vi "ChooseEstimation.vi"(6 "Time":enum16{"Azul", "Amarelo"}(ring) caption="Enum", 10 "Detection Frame Kalman":T1 {"robots_blue"."height" format="%+4.3f"; "robots_blue"."pixel_y" format="%+4.3f"; "robots_blue"."pixel_x" format="%+4.3f"; "robots_blue"."orientation" format="%+4.3f"; "robots_blue"."y" format="%+4.3f"; "robots_blue"."confidence" format="%4.3f"; "robots_blue"."x" format="%+4.3f"; "robots_yellow"."height" format="%+4.3f"; "robots_yellow"."pixel_y" format="%+4.3f"; "robots_yellow"."pixel_x" format="%+4.3f"; "robots_yellow"."orientation" format="%+4.3f"; "robots_yellow"."y" format="%+4.3f"; "robots_yellow"."confidence" format="%4.3f"; "robots_yellow"."x" format="%+4.3f"}, 11 "Detection Frame Kalman Vel Cmd":T1 {"robots_blue"."height" format="%+4.3f"; "robots_blue"."pixel_y" format="%+4.3f"; "robots_blue"."pixel_x" format="%+4.3f"; "robots_blue"."orientation" format="%+4.3f"; "robots_blue"."y" format="%+4.3f"; "robots_blue"."confidence" format="%4.3f"; "robots_blue"."x" format="%+4.3f"; "robots_yellow"."height" format="%+4.3f"; "robots_yellow"."pixel_y" format="%+4.3f"; "robots_yellow"."pixel_x" format="%+4.3f"; "robots_yellow"."orientation" format="%+4.3f"; "robots_yellow"."y" format="%+4.3f"; "robots_yellow"."confidence" format="%4.3f"; "robots_yellow"."x" format="%+4.3f"}) -> (2 "Detection Frame Out":T1 {"robots_blue"."height" format="%+4.3f"; "robots_blue"."pixel_y" format="%+4.3f"; "robots_blue"."pixel_x" format="%+4.3f"; "robots_blue"."orientation" format="%+4.3f"; "robots_blue"."y" format="%+4.3f"; "robots_blue"."confidence" format="%4.3f"; "robots_blue"."x" format="%+4.3f"; "robots_yellow"."height" format="%+4.3f"; "robots_yellow"."pixel_y" format="%+4.3f"; "robots_yellow"."pixel_x" format="%+4.3f"; "robots_yellow"."orientation" format="%+4.3f"; "robots_yellow"."y" format="%+4.3f"; "robots_yellow"."confidence" format="%4.3f"; "robots_yellow"."x" format="%+4.3f"})   [LabVIEW 2017]
uses:
  SSL Detection Frame.ctl
  SSL Detection Robot.ctl
  <vilib>/Analysis/Matrix/Datatypes/RealMatrix.ctl
  SSL Detection Ball.ctl
  <vilib>/Analysis/_algsub.llb/Real Vector Norm.vi
  <vilib>/ptbypt/NI_PtbyPt.lvlib
  <vilib>/Analysis/NI_AALPro.lvlib
  <vilib>/Analysis/Matrix/NI_Matrix.lvlib
panel:
  out "Enum":enum16{"Kalman Pure", "Kalman Vel Cmd"}(ring)
  out "norm 8":dbl
  out "norm 7":dbl
  out "norm 6":dbl
  out "norm 5":dbl
  out "Waveform Chart":cluster{"norm":dbl}(graph)
  out "norm 4":dbl
  out "norm 3":dbl
  out "norm 2":dbl
  out "norm":dbl
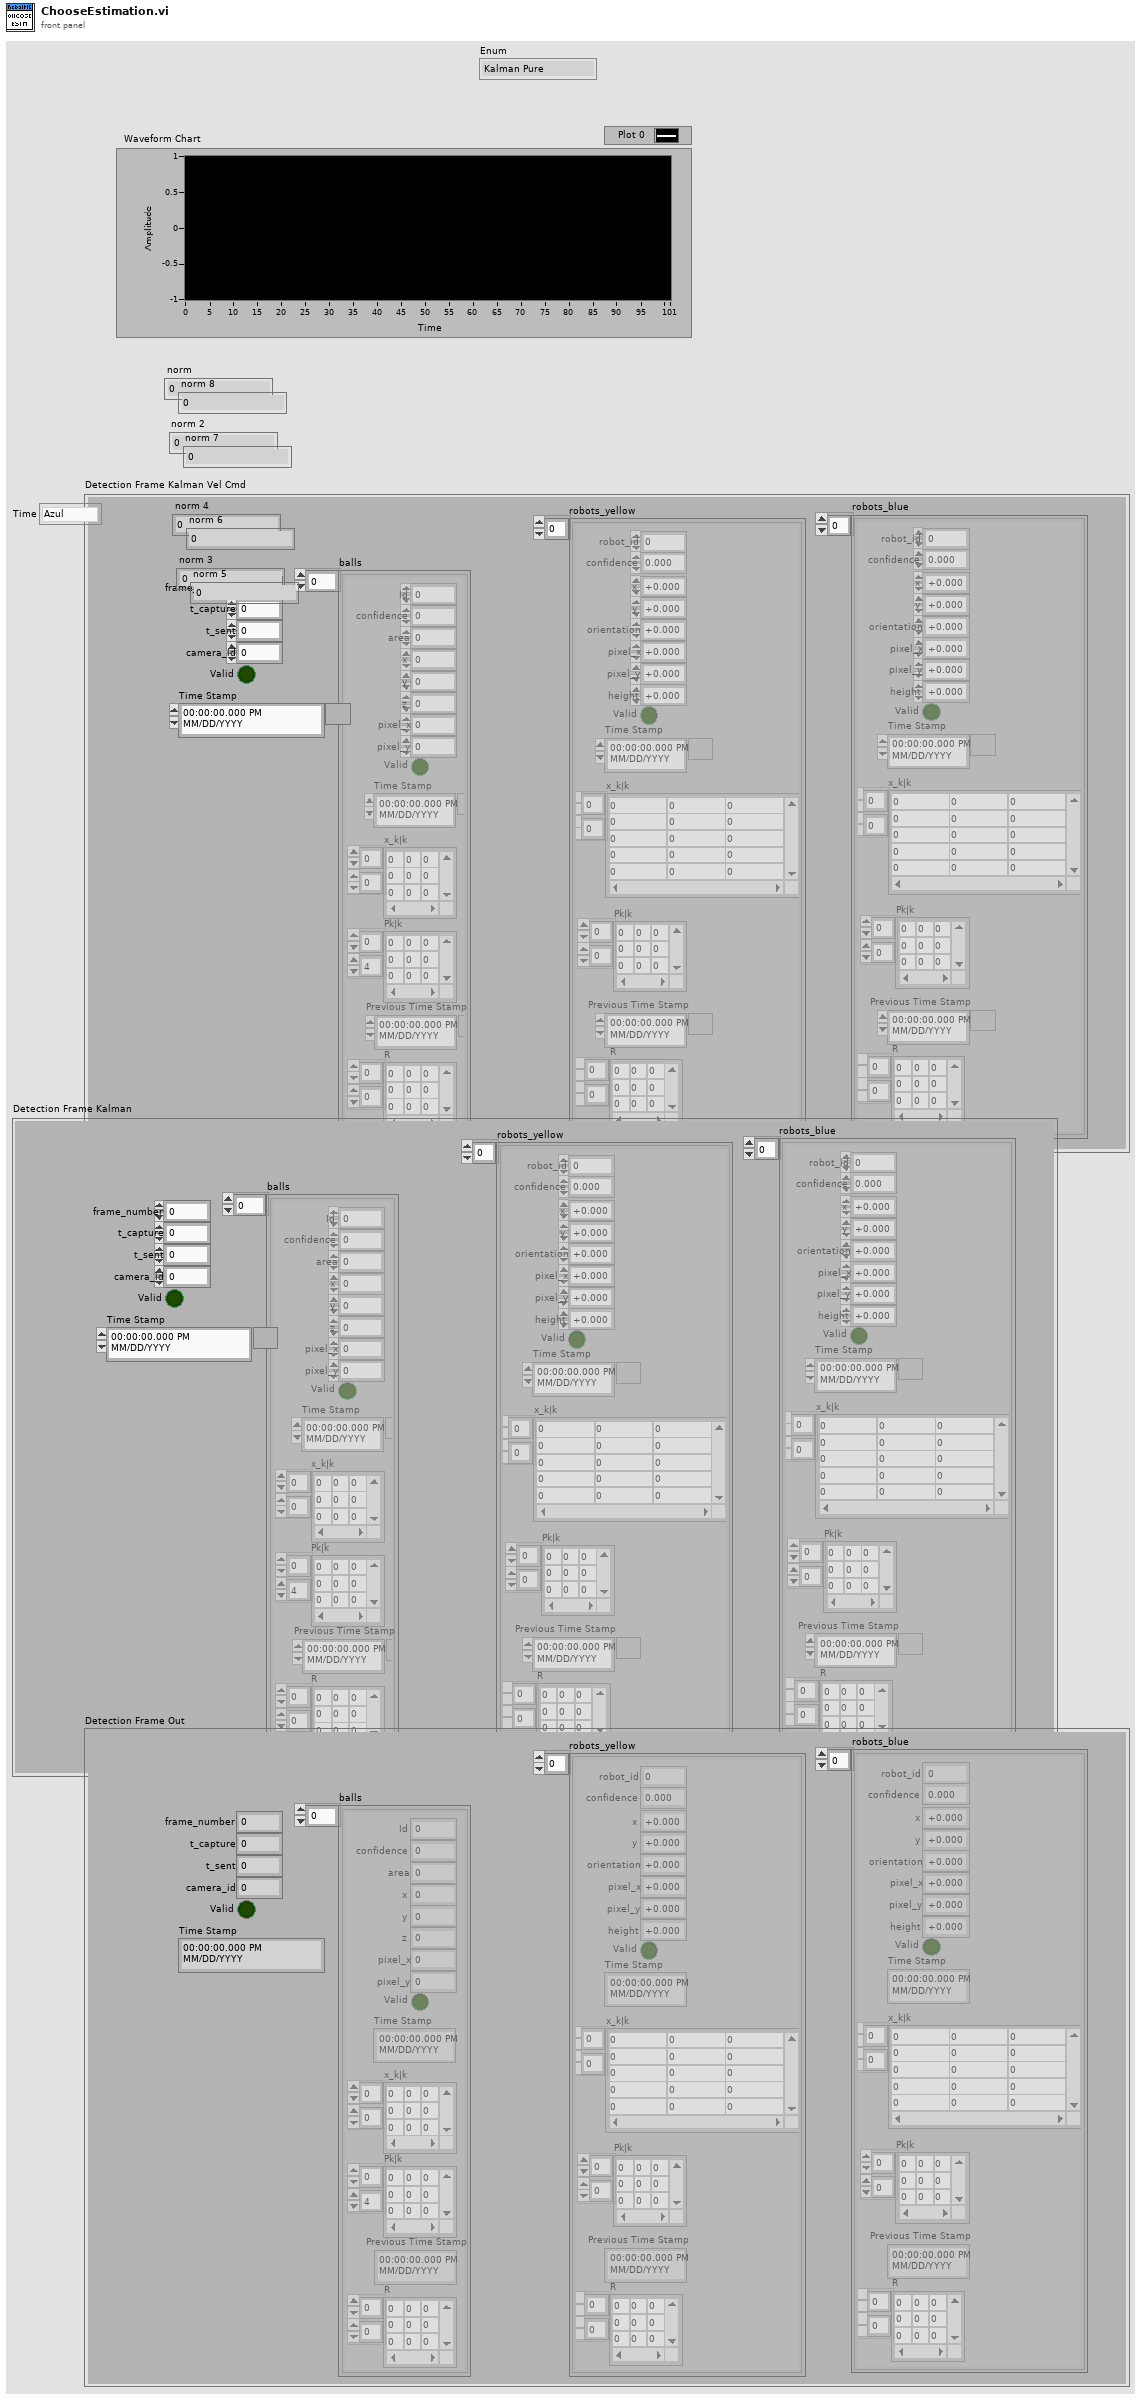
[diagram p1: front panel]
types:
  T1 = typedef "SSL Detection Frame.ctl" = cluster{"frame_number":u32, "t_capture":dbl, "t_sent":dbl, "camera_id":u32, "robots_yellow":T2[], "robots_blue":T2[], "balls":T4[], "Valid":bool, "Time Stamp":timestamp}
  T2 = typedef "SSL Detection Robot.ctl" = cluster{"x":sgl, "robot_id":u32, "confidence":sgl, "y":sgl, "orientation":sgl, "pixel_x":sgl, "pixel_y":sgl, "height":sgl, "Valid":bool, "Time Stamp":timestamp, "x_k|k":T3, "Pk|k":T3, "Previous Time Stamp":timestamp, "R":T3}
  T3 = typedef "NI_Matrix.lvlib/RealMatrix.ctl" = dbl[][]
  T4 = typedef "SSL Detection Ball.ctl" = cluster{"x":sgl, "area":u32, "confidence":sgl, "y":sgl, "z":sgl, "pixel_x":sgl, "pixel_y":sgl, "Valid":bool, "Time Stamp":timestamp, "x_k|k":T3, "Pk|k":T3, "Id":u32, "Previous Time Stamp":timestamp, "R":T3}
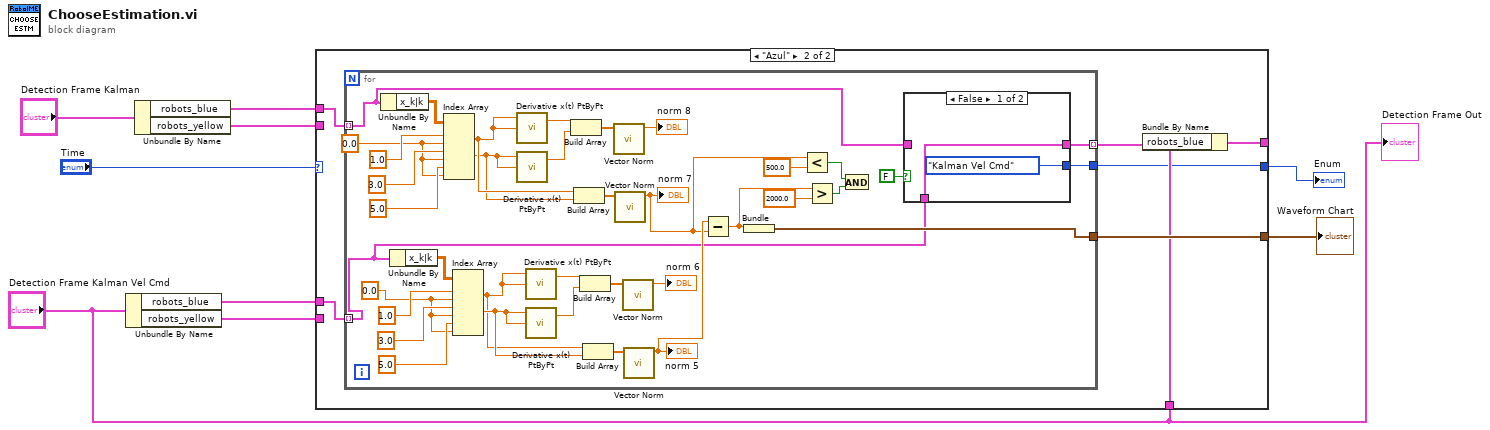
[diagram p0: block diagram]
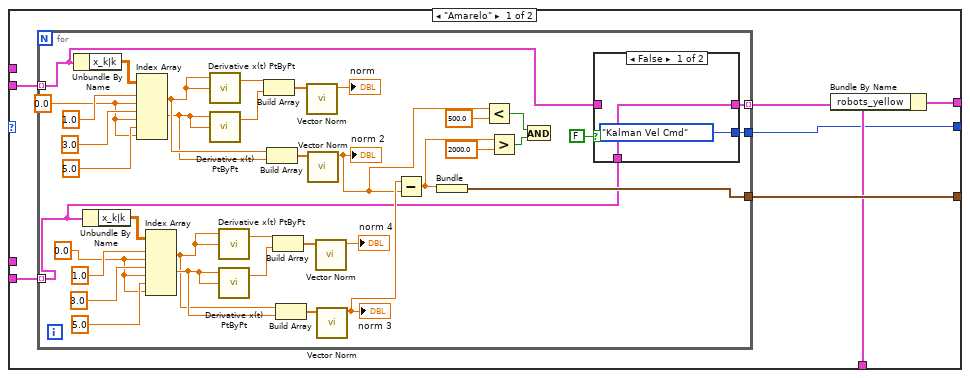
[diagram p2: hidden frame]
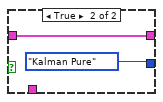
[diagram p3: hidden frame]
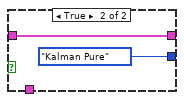
[diagram p4: hidden frame]
diagram:
  n1 = Unbundle By Name("Detection Frame Kalman Vel Cmd") -> ("robots_blue"=w4:T2[], "robots_yellow"=w6:T2[])
  n2 = Unbundle By Name("Detection Frame Kalman") -> ("robots_blue"=w3:T2[], "robots_yellow"=w8:T2[])
  n3 = case shown="\"Azul\"" "Time" {
    tunnel: w8 -> [w16 _]
    tunnel: w6 -> [w15 _]
    tunnel: [w14 w64] -> w5
    tunnel: "Detection Frame Kalman Vel Cmd" -> [w13 w63]
    tunnel: [w11 w61] -> _
    tunnel: w4 -> [_ w60]
    tunnel: w3 -> [_ w59]
    tunnel: [w10 w58] -> w2
    frame "Amarelo" {
      n4 = for {
        tunnel: w16 -> [w25] mode=indexing
        tunnel: w15 -> [w24] mode=indexing
        tunnel: [w30] -> w14
        tunnel: [w23] -> w12 mode=indexing
        tunnel: [w18] -> w10
        w32 = 0.0
        w50 = 0.0
        n5 = Unbundle By Name(w25) -> ("x_k|k"=w49:T3)
        n6 = Unbundle By Name(w24) -> ("x_k|k"=w36:T3)
        n7 = Index Array(array=w49, index (row) #1=1.0, index (col) #1=w50, index (row) #2=3.0, index (col) #2=w50, index (row) #3=5.0, index (col) #3=w50) -> (element #1=w45:dbl, element #2=w44:dbl)  [unwired: 1 out]
        n8 = Index Array(array=w36, index (row) #1=1.0, index (col) #1=w32, index (row) #2=3.0, index (col) #2=w32, index (row) #3=5.0, index (col) #3=w32) -> (element #1=w40:dbl, element #2=w41:dbl)  [unwired: 1 out]
        n9 = call <vilib>:"Derivative x(t) PtByPt.vi"("initial condition"=w45, "x"=w45) -> ("dx/dt"=w48:dbl)  [unwired: 2 in, 1 out]
        n10 = call <vilib>:"Derivative x(t) PtByPt.vi"("initial condition"=w44, "x"=w44) -> ("dx/dt"=w47:dbl)  [unwired: 2 in, 1 out]
        n11 = call <vilib>:"Derivative x(t) PtByPt.vi"("initial condition"=w40, "x"=w40) -> ("dx/dt"=w37:dbl)  [unwired: 2 in, 1 out]
        n12 = call <vilib>:"Derivative x(t) PtByPt.vi"("initial condition"=w41, "x"=w41) -> ("dx/dt"=w38:dbl)  [unwired: 2 in, 1 out]
        n13 = Build Array(w48, w47) -> (w46:dbl[])
        n14 = Build Array(w45, w44) -> (w43:dbl[])
        n15 = Build Array(w37, w38) -> (w39:dbl[])
        n16 = Build Array(w40, w41) -> (w42:dbl[])
        n17 = call-poly <vilib>:"Vector Norm.vi"("Input Vector"=w46) -> ("norm"=→"norm":dbl)  [unwired: 9 in, 1 out]
        n18 = call-poly <vilib>:"Vector Norm.vi"("Input Vector"=w43) -> ("norm"=w22:dbl)  [unwired: 9 in, 1 out]
        "norm 2" <- w22
        n19 = call-poly <vilib>:"Vector Norm.vi"("Input Vector"=w39) -> ("norm"=→"norm 4":dbl)  [unwired: 9 in, 1 out]
        n20 = call-poly <vilib>:"Vector Norm.vi"("Input Vector"=w42) -> ("norm"=w28:dbl)  [unwired: 9 in, 1 out]
        "norm 3" <- w28
        n21 = Subtract(x=w28, y=w22) -> (x-y=w27:dbl)
        n22 = Bundle(w27) -> (w30:cluster{dbl})  [unwired: 1 in]
        n23 = Less?(x=w22, y=500.0) -> (x < y?=w19:bool)
        n24 = Greater?(x=w27, y=2000.0) -> (0:w20:bool)
        n25 = And(x=w19, y=w20) -> ()  [unwired: 1 out]
        n26 = case shown="False" FALSE {
          tunnel: w25 -> [_ w57]
          tunnel: w24 -> [w55 _]
          tunnel: [w55 w57] -> w23
          tunnel: [enum16{"Kalman Pure", "Kalman Vel Cmd"}."Kalman Vel Cmd" ("Enum") enum16{"Kalman Pure", "Kalman Vel Cmd"}."Kalman Pure" ("Enum")] -> w18
          frame False {
          }
          frame True {
          }
        }
      }
      n27 = Bundle By Name(cluster=w13, "robots_yellow"=w12) -> (w11:T1)
    }
    frame "Azul" {
      n28 = for {
        tunnel: w59 -> [w75] mode=indexing
        tunnel: w60 -> [w74] mode=indexing
        tunnel: [w78] -> w64
        tunnel: [w73] -> w62 mode=indexing
        tunnel: [w72] -> w58
        w80 = 0.0
        w98 = 0.0
        n29 = Unbundle By Name(w75) -> ("x_k|k"=w97:T3)
        n30 = Unbundle By Name(w74) -> ("x_k|k"=w84:T3)
        n31 = Index Array(array=w97, index (row) #1=1.0, index (col) #1=w98, index (row) #2=3.0, index (col) #2=w98, index (row) #3=5.0, index (col) #3=w98) -> (element #1=w93:dbl, element #2=w92:dbl)  [unwired: 1 out]
        n32 = Index Array(array=w84, index (row) #1=1.0, index (col) #1=w80, index (row) #2=3.0, index (col) #2=w80, index (row) #3=5.0, index (col) #3=w80) -> (element #1=w88:dbl, element #2=w89:dbl)  [unwired: 1 out]
        n33 = call <vilib>:"Derivative x(t) PtByPt.vi"("initial condition"=w93, "x"=w93) -> ("dx/dt"=w96:dbl)  [unwired: 2 in, 1 out]
        n34 = call <vilib>:"Derivative x(t) PtByPt.vi"("initial condition"=w92, "x"=w92) -> ("dx/dt"=w95:dbl)  [unwired: 2 in, 1 out]
        n35 = call <vilib>:"Derivative x(t) PtByPt.vi"("initial condition"=w88, "x"=w88) -> ("dx/dt"=w85:dbl)  [unwired: 2 in, 1 out]
        n36 = call <vilib>:"Derivative x(t) PtByPt.vi"("initial condition"=w89, "x"=w89) -> ("dx/dt"=w86:dbl)  [unwired: 2 in, 1 out]
        n37 = Build Array(w96, w95) -> (w94:dbl[])
        n38 = Build Array(w93, w92) -> (w91:dbl[])
        n39 = Build Array(w85, w86) -> (w87:dbl[])
        n40 = Build Array(w88, w89) -> (w90:dbl[])
        n41 = call-poly <vilib>:"Vector Norm.vi"("Input Vector"=w94) -> ("norm"=→"norm 8":dbl)  [unwired: 9 in, 1 out]
        n42 = call-poly <vilib>:"Vector Norm.vi"("Input Vector"=w91) -> ("norm"=w67:dbl)  [unwired: 9 in, 1 out]
        "norm 7" <- w67
        n43 = call-poly <vilib>:"Vector Norm.vi"("Input Vector"=w87) -> ("norm"=→"norm 6":dbl)  [unwired: 9 in, 1 out]
        n44 = call-poly <vilib>:"Vector Norm.vi"("Input Vector"=w90) -> ("norm"=w76:dbl)  [unwired: 9 in, 1 out]
        "norm 5" <- w76
        n45 = Subtract(x=w76, y=w67) -> (x-y=w66:dbl)
        n46 = Bundle(w66) -> (w78:cluster{dbl})  [unwired: 1 in]
        n47 = Less?(x=w67, y=500.0) -> (x < y?=w68:bool)
        n48 = Greater?(x=w66, y=2000.0) -> (0:w69:bool)
        n49 = And(x=w68, y=w69) -> ()  [unwired: 1 out]
        n50 = case shown="False" FALSE {
          tunnel: w75 -> [_ w105]
          tunnel: w74 -> [w103 _]
          tunnel: [w103 w105] -> w73
          tunnel: [enum16{"Kalman Pure", "Kalman Vel Cmd"}."Kalman Vel Cmd" ("Enum") enum16{"Kalman Pure", "Kalman Vel Cmd"}."Kalman Pure" ("Enum")] -> w72
          frame False {
          }
          frame True {
          }
        }
      }
      n51 = Bundle By Name(cluster=w63, "robots_blue"=w62) -> (w61:T1)
    }
  }
  "Waveform Chart" <- w5
  "Enum" <- w2
  "Detection Frame Out" <- "Detection Frame Kalman Vel Cmd"
